vi "ObjectFactory.vi"(0 "GOject":refnum<vi>, 5 "error in (no error)":errorcluster) -> (14 "Object":refnum<class "Object.lvclass">, 15 "Is Indicator":bool, 16 "Is Control":bool, 17 "Is Visible":bool, 19 "error out":errorcluster)   [LabVIEW 2014, in "WebFrontPanel.lvclass"]
doc: "Convert FP refs into \"HTML\" objects"
uses:
  WebFrontPanel.lvclass
  Object_class/Object.lvclass
  Object_class/Attributes.ctl
  Object_class/Coordinates.ctl
  Control_class/Attributes.ctl
  Text_class/Text.lvclass
  BooleanControl_class/Attributes.ctl
  Numeric_class/Attributes.ctl
  String_class/Attributes.ctl
  Graph_class/Attributes.ctl
  Select_class/Attributes.ctl
  Progressbar_class/Attributes.ctl
  Text_class/Attributes.ctl
  Control_class/Control.lvclass
  BooleanControl_class/BooleanControl.lvclass
  Graph_class/Graph.lvclass
  Numeric_class/Numeric.lvclass
  String_class/String.lvclass
  Select_class/Select.lvclass
  Progressbar_class/Progressbar.lvclass
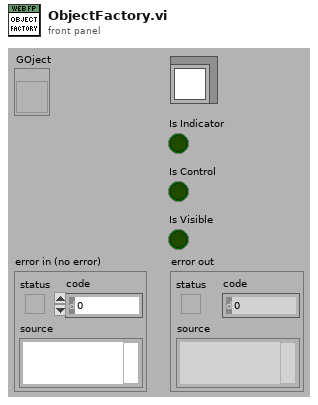
[diagram p1: front panel]
types:
  T1 = typedef "Object.lvclass/Attributes.ctl" = cluster{"UID":i32, "Type":string, "Coordinates":T2, "Reference":refnum<vi>}
  T2 = typedef "Object.lvclass/Coordinates.ctl" = cluster{"Left":i32, "Top":i32, "Height":u32, "Width":u32}
  T3 = typedef "Control.lvclass/Attributes.ctl" = cluster{"Description":string, "Indicator":bool, "Default Value":variant, "Control Index":i32, "Label":refnum<class "Text.lvclass">, "Caption":refnum<class "Text.lvclass">, "Use Picture":bool, "Image1 b64":string, "Image2 b64":string}
  T4 = typedef "BooleanControl.lvclass/Attributes.ctl" = cluster{"Boolean ref":refnum<vi>, "Switching":bool, "Boolean Strings":string[], "Text":refnum<class "Text.lvclass">}
  T5 = typedef "Numeric.lvclass/Attributes.ctl" = cluster{"unused":dbl}
  T6 = typedef "String.lvclass/Attributes.ctl" = cluster{"unused":string}
  T7 = typedef "Graph.lvclass/Attributes.ctl" = cluster{"not used":dbl}
  T8 = typedef "Select.lvclass/Attributes.ctl" = cluster{"not used":dbl}
  T9 = typedef "Progressbar.lvclass/Attributes.ctl" = cluster{"not used":dbl}
  T10 = cluster{"Object":T1, "Control":T3, "Boolean":T4, "Numeric":T5, "String":T6, "Graph":T7, "Select":T8, "Progressbar":T9, "Object out":refnum<class "Object.lvclass">, "Label":refnum<class "Text.lvclass">, "Caption":refnum<class "Text.lvclass">, "Is Indicator":bool, "Is Control":bool, "Is Visible":bool}
  T11 = typedef "Text.lvclass/Attributes.ctl" = cluster{"Text":string, "Font":string, "Font Size":u32, "Visible":bool}
  T12 = typedef "LVRectTypeDef.ctl" = cluster{"Left":i16, "Top":i16, "Right":i16, "Bottom":i16}
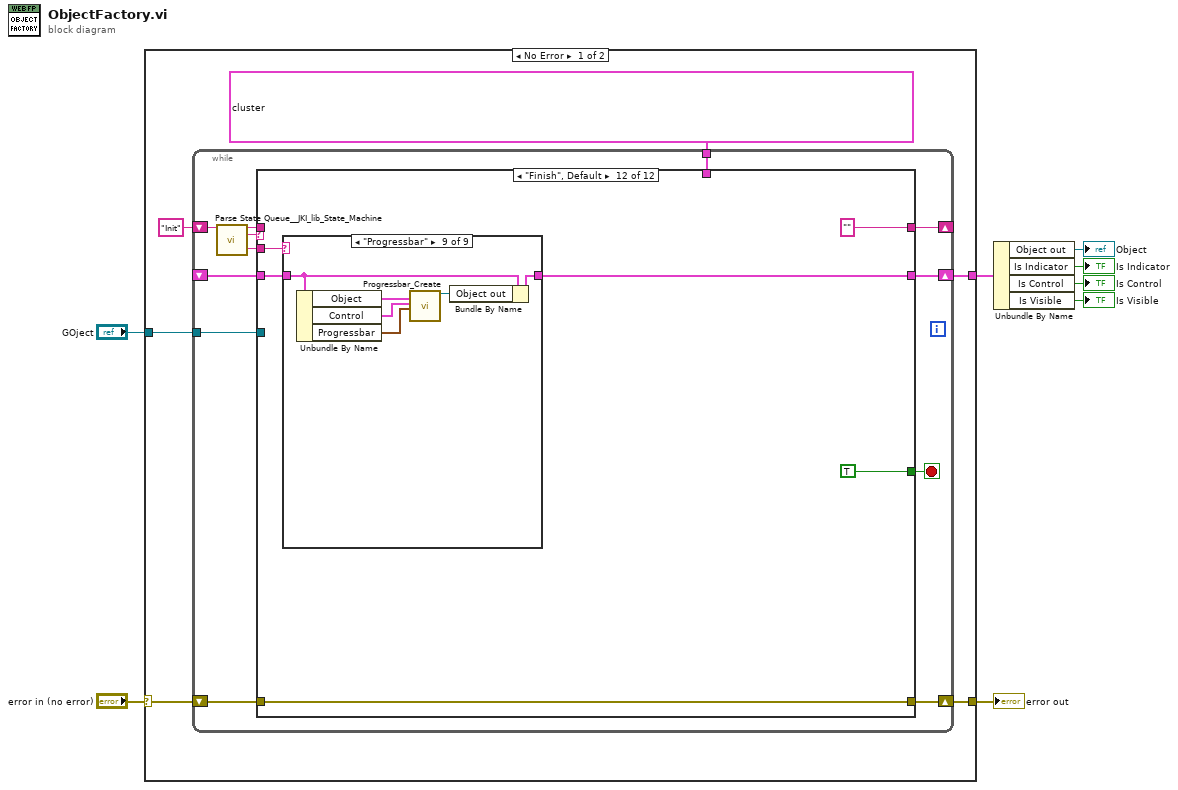
[diagram p0: block diagram]
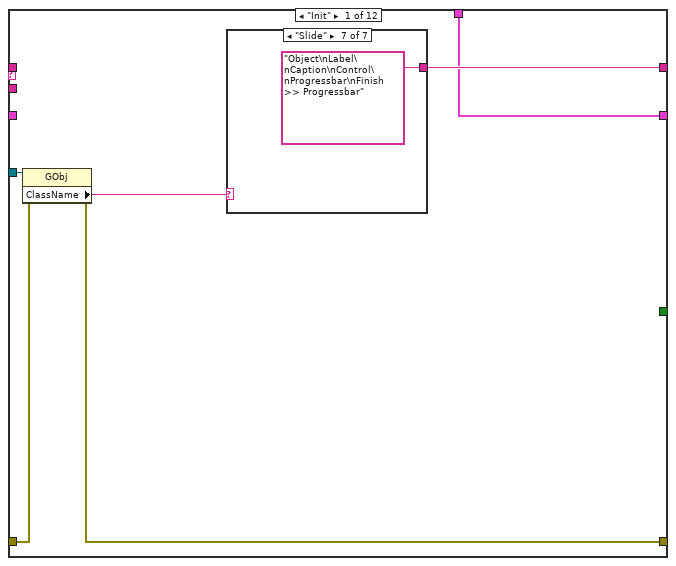
[diagram p2: hidden frame]
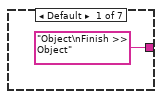
[diagram p3: hidden frame]
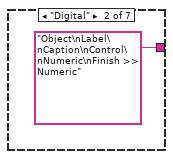
[diagram p4: hidden frame]
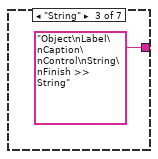
[diagram p5: hidden frame]
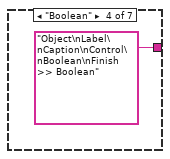
[diagram p6: hidden frame]
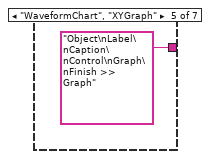
[diagram p7: hidden frame]
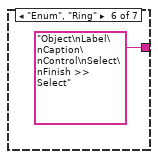
[diagram p8: hidden frame]
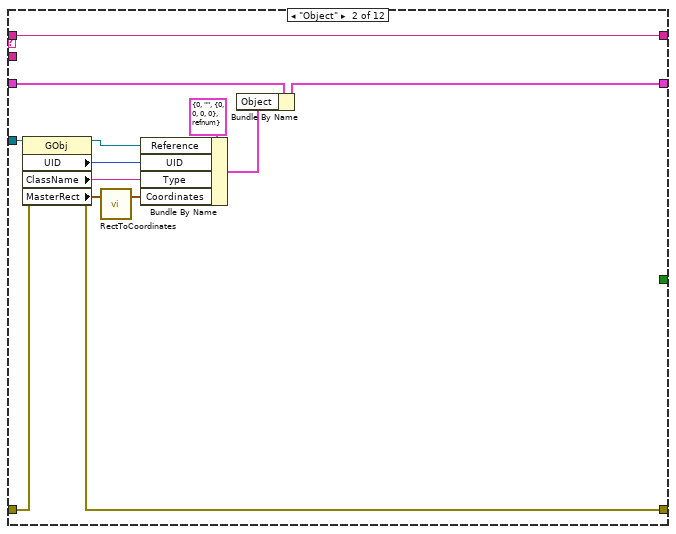
[diagram p9: hidden frame]
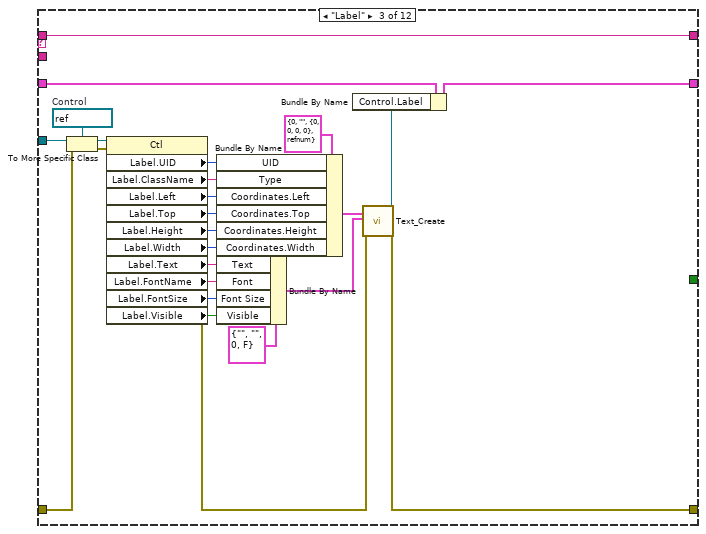
[diagram p10: hidden frame]
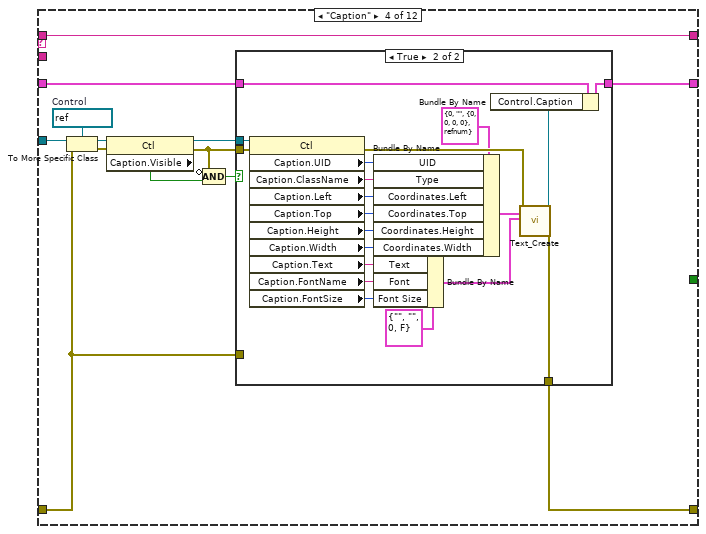
[diagram p11: hidden frame]
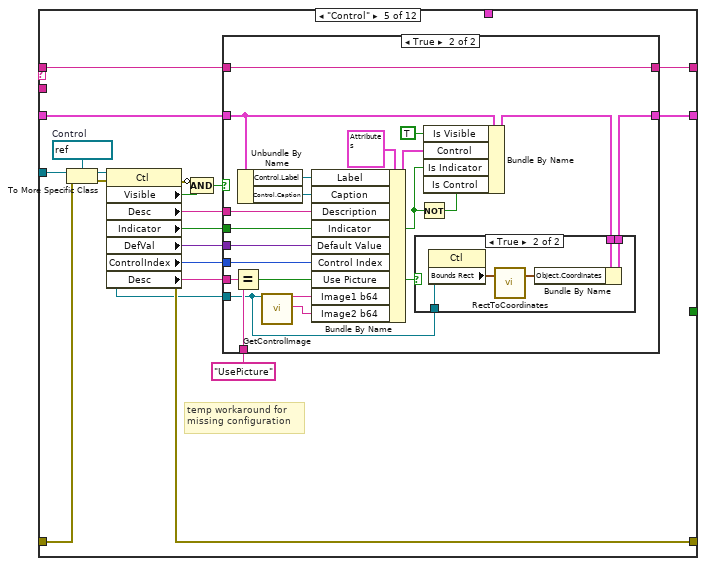
[diagram p13: hidden frame]
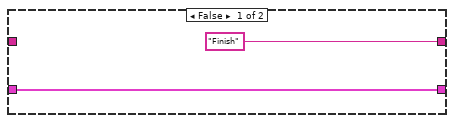
[diagram p14: hidden frame]
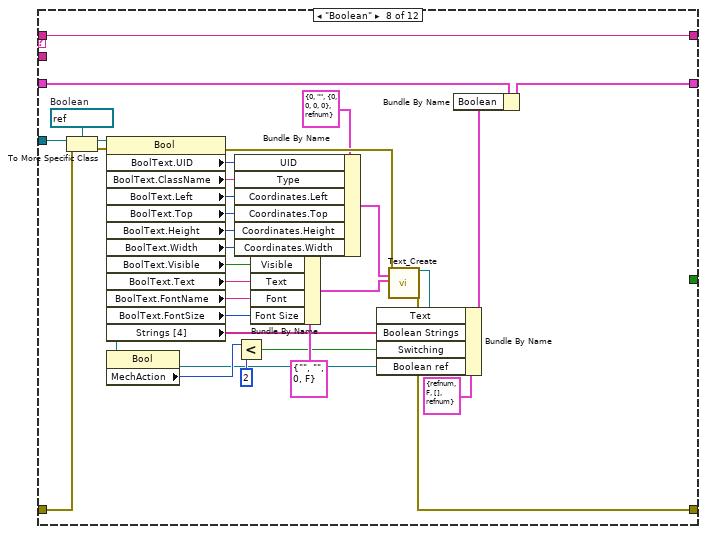
[diagram p18: hidden frame]
diagram:
  n1 = case shown="No Error" "error in (no error)" {
    selector: "error in (no error)" -> [w13 w257]
    tunnel: [w14 w257] -> w7
    tunnel: "GOject" -> [w12 _]
    tunnel: [w9 _] -> w5
    frame No Error {
      n2 = while {
        tunnel: w12 -> [w24]
        shift-right: [w15] -> _
        shift-left: "Init" -> [w19]
        shift-right: [w23] -> w9
        shift-left: _ -> [w22]
        shift-right: [w25] -> w14
        shift-left: w13 -> [w26]
        tunnel: T10 {"Object"={"UID"=0, "Type"="", "Coordinates"={"Left"=0, "Top"=0, "Height"=0, "Width"=0}, "Reference"=refnum}, "Control"={"Description"="", "Indicator"=FALSE, "Default Value"=variant, "Control Index"=0, "Label"=refnum, "Caption"=refnum, "Use Picture"=FALSE, "Image1 b64"="", "Image2 b64"=""}, "Boolean"={"Boolean ref"=refnum, "Switching"=FALSE, "Boolean Strings"=[], "Text"=refnum}, "Numeric"={"unused"=0.0}, "String"={"unused"=""}, "Graph"={"not used"=0.0}, "Select"={"not used"=0.0}, "Progressbar"={"not used"=0.0}, "Object out"=refnum, "Label"=refnum, "Caption"=refnum, "Is Indicator"=FALSE, "Is Control"=FALSE, "Is Visible"=FALSE} -> [w21]
        stop <- w20 stop-if-true
        n3 = call <vilib>:"Parse State Queue__JKI_lib_State_Machine.vi"("State Queue"=w19) -> ("Remaining States"=w16:string, "Current State"=w18:string, "Arguments"=w17:string)  [unwired: 12 in]
        n4 = case shown="\"Finish\", Default" w18 {
          tunnel: w24 -> [w30 w48 w72 w84 w126 _ _ w192 _ _ _ _]
          tunnel: [w28 w45 w60 w79 w117 w161 w164 w189 w198 w201 w204 ""] -> w15
          tunnel: [w27 w47 w61 w80 w120 w160 w163 w190 w196 w199 w202 w206] -> w23
          tunnel: w22 -> [_ w46 w62 w81 w125 w160 w163 w191 w196 w199 w202 w205]
          tunnel: [w31 w51 w75 w88 w128 w159 w162 w195 w197 w200 w203 w210] -> w25
          tunnel: w26 -> [w32 w52 w76 w87 w129 w159 w162 w194 w197 w200 w203 w210]
          tunnel: w21 -> [w27 _ _ _ _ _ _ _ _ _ _ _]
          tunnel: [_ _ _ _ _ _ _ _ _ _ _ TRUE] -> w20
          tunnel: w17 -> [_ _ _ _ _ _ _ _ _ _ _ w207]
          tunnel: w16 -> [_ w45 w60 w79 w116 w161 w164 w189 w198 w201 w204 _]
          frame "Init" {
            n5 = property class="GObj"(reference=w30, error in=w32) -> (error out=w31:errorcluster, "ClassName"=w29:string)  [unwired: 1 out]
            n6 = case shown="\"Slide\"" w29 {
              tunnel: ["Object\nFinish >> Object" "Object\nLabel\nCaption\nControl\nNumeric\nFinish >> Numeric" "Object\nLabel\nCaption\nControl\nString\nFinish >> String" "Object\nLabel\nCaption\nControl\nBoolean\nFinish >> Boolean" "Object\nLabel\nCaption\nControl\nGraph\nFinish >> Graph" "Object\nLabel\nCaption\nControl\nSelect\nFinish >> Select" "Object\nLabel\nCaption\nControl\nProgressbar\nFinish >> Progressbar"] -> w28
              frame Default {
              }
              frame "Digital" {
              }
              frame "String" {
              }
              frame "Boolean" {
              }
              frame "WaveformChart", "XYGraph" {
              }
              frame "Enum", "Ring" {
              }
              frame "Slide" {
              }
            }
          }
          frame "Object" {
            n7 = property class="GObj"(reference=w48, error in=w52) -> (reference out=w40:refnum<vi>, error out=w51:errorcluster, "UID"=w49:i32, "ClassName"=w50:string, "MasterRect"=w42:T12)
            n8 = call "RectToCoordinates.vi"("Rect"=w42) -> ("Coordinates"=w41:T2)  [unwired: 2 in]
            n9 = Bundle By Name(cluster=T1 {"UID"=0, "Type"="", "Coordinates"={"Left"=0, "Top"=0, "Height"=0, "Width"=0}, "Reference"=refnum} ("Object Attributes"), "Reference"=w40, "UID"=w49, "Type"=w50, "Coordinates"=w41) -> (w43:T1)
            n10 = Bundle By Name(cluster=w46, "Object"=w43) -> (w47:T10)
          }
          frame "Label" {
            w74 = refnum<vi> refnum  # Control
            n11 = To More Specific Class(target class=w74, reference=w72, error in=w76) -> (specific class reference=w73:refnum<vi>, error out=w77:errorcluster)
            n12 = property class="Ctl"(reference=w73, error in=w77) -> (error out=w54:errorcluster, "Label.UID"=w71:i32, "Label.ClassName"=w70:string, "Label.Left"=w69:i32, "Label.Top"=w68:i32, "Label.Height"=w67:u32, "Label.Width"=w66:u32, "Label.Text"=w65:string, "Label.FontName"=w64:string, "Label.FontSize"=w63:u32, "Label.Visible"=w53:bool)  [unwired: 1 out]
            n13 = Bundle By Name(cluster=T1 {"UID"=0, "Type"="", "Coordinates"={"Left"=0, "Top"=0, "Height"=0, "Width"=0}, "Reference"=refnum} ("Object Attributes"), "UID"=w71, "Type"=w70, "Coordinates.Left"=w69, "Coordinates.Top"=w68, "Coordinates.Height"=w67, "Coordinates.Width"=w66) -> (w57:T1)
            n14 = Bundle By Name(cluster=T11 {"Text"="", "Font"="", "Font Size"=0, "Visible"=FALSE} ("Text Attributes"), "Text"=w65, "Font"=w64, "Font Size"=w63, "Visible"=w53) -> (w56:T11)
            n15 = call "Text_Create.vi"("Object Attributes"=w57, "Text Attributes"=w56, "error in (no error)"=w54) -> ("reference out"=w55:refnum<class "Text.lvclass">, "error out"=w75:errorcluster)  [unwired: 15 in]
            n16 = Bundle By Name(cluster=w62, "Control.Label"=w55) -> (w61:T10)
          }
          frame "Caption" {
            w86 = refnum<vi> refnum  # Control
            n17 = To More Specific Class(target class=w86, reference=w84, error in=w87) -> (specific class reference=w85:refnum<vi>, error out=w90:errorcluster)
            n18 = property class="Ctl"(reference=w85, error in=w90) -> (reference out=w78:refnum<vi>, error out=w89:errorcluster, "Caption.Visible"=w83:bool)
            n19 = Compound Arithmetic op=AND(invert w89, w83) -> (w82:bool)
            n20 = case shown="True" w82 {
              tunnel: w81 -> [w91 w105]
              tunnel: [w91 w104] -> w80
              tunnel: w78 -> [_ w102]
              tunnel: w89 -> [_ w112]
              tunnel: [w92 w110] -> w88
              tunnel: w87 -> [w92 _]
              frame False {
              }
              frame True {
                n21 = property class="Ctl"(reference=w102, error in=w112) -> (error out=w111:errorcluster, "Caption.UID"=w101:i32, "Caption.ClassName"=w100:string, "Caption.Left"=w99:i32, "Caption.Top"=w98:i32, "Caption.Height"=w97:u32, "Caption.Width"=w96:u32, "Caption.Text"=w95:string, "Caption.FontName"=w94:string, "Caption.FontSize"=w93:u32)  [unwired: 1 out]
                n22 = Bundle By Name(cluster=T1 {"UID"=0, "Type"="", "Coordinates"={"Left"=0, "Top"=0, "Height"=0, "Width"=0}, "Reference"=refnum} ("Object Attributes"), "UID"=w101, "Type"=w100, "Coordinates.Left"=w99, "Coordinates.Top"=w98, "Coordinates.Height"=w97, "Coordinates.Width"=w96) -> (w107:T1)
                n23 = Bundle By Name(cluster=T11 {"Text"="", "Font"="", "Font Size"=0, "Visible"=FALSE} ("Text Attributes"), "Text"=w95, "Font"=w94, "Font Size"=w93) -> (w106:T11)
                n24 = call "Text_Create.vi"("Object Attributes"=w107, "Text Attributes"=w106, "error in (no error)"=w111) -> ("reference out"=w103:refnum<class "Text.lvclass">, "error out"=w110:errorcluster)  [unwired: 15 in]
                n25 = Bundle By Name(cluster=w105, "Control.Caption"=w103) -> (w104:T10)
              }
            }
          }
          frame "Control" {
            w127 = refnum<vi> refnum  # Control
            # "temp workaround for\nmissing configuration"
            n26 = To More Specific Class(target class=w127, reference=w126, error in=w129) -> (specific class reference=w114:refnum<vi>, error out=w130:errorcluster)
            n27 = property class="Ctl"(reference=w114, error in=w130) -> (error out=w128:errorcluster, "Visible"=w118:bool, "Desc"=w124:string, "Indicator"=w123:bool, "DefVal"=w122:variant, "ControlIndex"=w121:i32, "Desc"=w113:string)  [unwired: 1 out]
            n28 = Compound Arithmetic op=AND(invert w128, w118) -> (w119:bool)
            n29 = case shown="True" w119 {
              tunnel: w125 -> [w132 w146]
              tunnel: w124 -> [_ w152]
              tunnel: w123 -> [_ w142]
              tunnel: w122 -> [_ w151]
              tunnel: w121 -> [_ w150]
              tunnel: [w132 w135] -> w120
              tunnel: ["Finish" w147] -> w117
              tunnel: w116 -> [_ w147]
              tunnel: "UsePicture" -> [_ w140]
              tunnel: w114 -> [_ w133]
              tunnel: w113 -> [_ w137]
              frame False {
              }
              frame True {
                n30 = Equal?(x=w137, y=w140) -> (x = y?=w134:bool)
                n31 = Unbundle By Name(w146) -> ("Control.Label"=w145:refnum<class "Text.lvclass">, "Control.Caption"=w144:refnum<class "Text.lvclass">)
                n32 = call "GetControlImage.vi"("Control ref"=w133) -> ("base64 encoded <img> string 1"=w139:string, "base64 encoded <img> string 2"=w138:string)  [unwired: 16 in, 1 out]
                n33 = Bundle By Name(cluster=T3 {"Description"="", "Indicator"=FALSE, "Default Value"=variant, "Control Index"=0, "Label"=refnum, "Caption"=refnum, "Use Picture"=FALSE, "Image1 b64"="", "Image2 b64"=""} ("Control Attributes"), "Label"=w145, "Caption"=w144, "Description"=w152, "Indicator"=w142, "Default Value"=w151, "Control Index"=w150, "Use Picture"=w134, "Image1 b64"=w139, "Image2 b64"=w138) -> (w148:T3)
                n34 = Not(x=w142) -> (.not. x?=w141:bool)
                n35 = Bundle By Name(cluster=w146, "Is Visible"=TRUE, "Control"=w148, "Is Indicator"=w142, "Is Control"=w141) -> (w136:T10)
                n36 = case shown="True" w134 {
                  tunnel: w136 -> [w153 w158]
                  tunnel: [w153 w157] -> w135
                  tunnel: w133 -> [_ w156]
                  frame False {
                  }
                  frame True {
                    n37 = property class="Ctl"(reference=w156) -> ("Bounds Rect"=w155:T12)  [unwired: 1 in, 2 out]
                    n38 = call "RectToCoordinates.vi"("Rect"=w155) -> ("Coordinates"=w154:T2)  [unwired: 2 in]
                    n39 = Bundle By Name(cluster=w158, "Object.Coordinates"=w154) -> (w157:T10)
                  }
                }
              }
            }
          }
          frame "Numeric" {
            # "All properties are queried at run time"
          }
          frame "String" {
            # "All properties are queried at run time"
          }
          frame "Boolean" {
            w193 = refnum<vi> refnum  # Boolean
            n40 = To More Specific Class(target class=w193, reference=w192, error in=w194) -> (specific class reference=w165:refnum<vi>, error out=w167:errorcluster)
            n41 = property class="Bool"(reference=w165, error in=w167) -> (error out=w188:errorcluster, "BoolText.UID"=w178:i32, "BoolText.ClassName"=w177:string, "BoolText.Left"=w176:i32, "BoolText.Top"=w175:i32, "BoolText.Height"=w174:u32, "BoolText.Width"=w173:u32, "BoolText.Visible"=w168:bool, "BoolText.Text"=w172:string, "BoolText.FontName"=w171:string, "BoolText.FontSize"=w170:u32, "Strings [4]"=w169:string[])  [unwired: 1 out]
            n42 = property class="Bool"(reference=w165) -> ("MechAction"=w166:u32)  [unwired: 1 in, 2 out]
            n43 = Bundle By Name(cluster=T1 {"UID"=0, "Type"="", "Coordinates"={"Left"=0, "Top"=0, "Height"=0, "Width"=0}, "Reference"=refnum} ("Object Attributes"), "UID"=w178, "Type"=w177, "Coordinates.Left"=w176, "Coordinates.Top"=w175, "Coordinates.Height"=w174, "Coordinates.Width"=w173) -> (w183:T1)
            n44 = Less?(x=w166, y=u32 2) -> (x < y?=w179:bool)
            n45 = Bundle By Name(cluster=T11 {"Text"="", "Font"="", "Font Size"=0, "Visible"=FALSE} ("Text Attributes"), "Visible"=w168, "Text"=w172, "Font"=w171, "Font Size"=w170) -> (w182:T11)
            n46 = call "Text_Create.vi"("Object Attributes"=w183, "Text Attributes"=w182, "error in (no error)"=w188) -> ("reference out"=w181:refnum<class "Text.lvclass">, "error out"=w195:errorcluster)  [unwired: 15 in]
            n47 = Bundle By Name(cluster=T4 {"Boolean ref"=refnum, "Switching"=FALSE, "Boolean Strings"=[], "Text"=refnum} ("BooleanControl Attributes"), "Text"=w181, "Boolean Strings"=w169, "Switching"=w179, "Boolean ref"=w165) -> (w180:T4)
            n48 = Bundle By Name(cluster=w191, "Boolean"=w180) -> (w190:T10)
          }
          frame "Graph" {
            # "All properties are queried at run time"
          }
          frame "Select" {
            # "All properties are queried at run time"
          }
          frame "Progressbar" {
            # "All properties are queried at run time"
          }
          frame "Finish", Default {
            n49 = case shown="\"Progressbar\"" w207 {
              tunnel: [w211 w213 w219 w222 w230 w236 w242 w248 w254] -> w206
              tunnel: w205 -> [w211 w215 w220 w226 w232 w238 w244 w250 w256]
              frame Default {
              }
              frame "Object" {
                n50 = Unbundle By Name(w215) -> ("Object"=w214:T1)
                n51 = call "Object_Create.vi"("Object Attributes"=w214) -> ("reference out"=w212:refnum<class "Object.lvclass">)  [unwired: 17 in, 1 out]
                n52 = Bundle By Name(cluster=w215, "Object out"=w212) -> (w213:T10)
              }
              frame "Control" {
                n53 = Unbundle By Name(w220) -> ("Object"=w217:T1, "Control"=w216:T3)
                n54 = call "Control_Create.vi"("Object Attributes"=w217, "Control Attributes"=w216) -> ("reference out"=w218:refnum<class "Control.lvclass">)  [unwired: 16 in, 1 out]
                n55 = Bundle By Name(cluster=w220, "Object out"=w218) -> (w219:T10)
              }
              frame "Boolean" {
                n56 = Unbundle By Name(w226) -> ("Object"=w225:T1, "Control"=w224:T3, "Boolean"=w223:T4)
                n57 = call "BooleanControl_Create.vi"("Object Attributes"=w225, "Control Attributes"=w224, "BooleanControl Attributes"=w223) -> ("reference out"=w221:refnum<class "BooleanControl.lvclass">)  [unwired: 15 in, 1 out]
                n58 = Bundle By Name(cluster=w226, "Object out"=w221) -> (w222:T10)
              }
              frame "Graph" {
                n59 = Unbundle By Name(w232) -> ("Object"=w228:T1, "Control"=w231:T3, "Graph"=w227:T7)
                n60 = call "Graph_Create.vi"("Object Attributes"=w228, "Control Attributes"=w231, "Graph Attributes"=w227) -> ("reference out"=w229:refnum<class "Graph.lvclass">)  [unwired: 15 in, 1 out]
                n61 = Bundle By Name(cluster=w232, "Object out"=w229) -> (w230:T10)
              }
              frame "Numeric" {
                n62 = Unbundle By Name(w238) -> ("Object"=w234:T1, "Control"=w237:T3, "Numeric"=w233:T5)
                n63 = call "Numeric_Create.vi"("Object Attributes"=w234, "Control Attributes"=w237, "Graph Attributes"=w233) -> ("reference out"=w235:refnum<class "Numeric.lvclass">)  [unwired: 15 in, 1 out]
                n64 = Bundle By Name(cluster=w238, "Object out"=w235) -> (w236:T10)
              }
              frame "String" {
                n65 = Unbundle By Name(w244) -> ("Object"=w240:T1, "Control"=w243:T3, "String"=w239:T6)
                n66 = call "String_Create.vi"("Object Attributes"=w240, "Control Attributes"=w243, "String Attributes"=w239) -> ("reference out"=w241:refnum<class "String.lvclass">)  [unwired: 15 in, 1 out]
                n67 = Bundle By Name(cluster=w244, "Object out"=w241) -> (w242:T10)
              }
              frame "Select" {
                n68 = Unbundle By Name(w250) -> ("Object"=w246:T1, "Control"=w249:T3, "Select"=w245:T8)
                n69 = call "Select_Create.vi"("Object Attributes"=w246, "Control Attributes"=w249, "Select Attributes"=w245) -> ("reference out"=w247:refnum<class "Select.lvclass">)  [unwired: 15 in, 1 out]
                n70 = Bundle By Name(cluster=w250, "Object out"=w247) -> (w248:T10)
              }
              frame "Progressbar" {
                n71 = Unbundle By Name(w256) -> ("Object"=w252:T1, "Control"=w255:T3, "Progressbar"=w251:T9)
                n72 = call "Progressbar_Create.vi"("Object Attributes"=w252, "Control Attributes"=w255, "Progressbar Attributes"=w251) -> ("reference out"=w253:refnum<class "Progressbar.lvclass">)  [unwired: 15 in, 1 out]
                n73 = Bundle By Name(cluster=w256, "Object out"=w253) -> (w254:T10)
              }
            }
          }
        }
      }
    }
    frame Error {
    }
  }
  "error out" <- w7
  n74 = Unbundle By Name(w5) -> ("Object out"=→"Object":refnum<class "Object.lvclass">, "Is Indicator"=→"Is Indicator":bool, "Is Control"=→"Is Control":bool, "Is Visible"=→"Is Visible":bool)
